vi "TestAddConpane.vi"() -> ()   [LabVIEW 2015]
uses:
  <vilib>/Utility/miscctls.llb/LVPositionTypeDef.ctl
panel:
  in  "E F":dbl
  in  "E":dbl
  in  "D":dbl
  in  "C":dbl
  in  "B":dbl
  in  "A":dbl
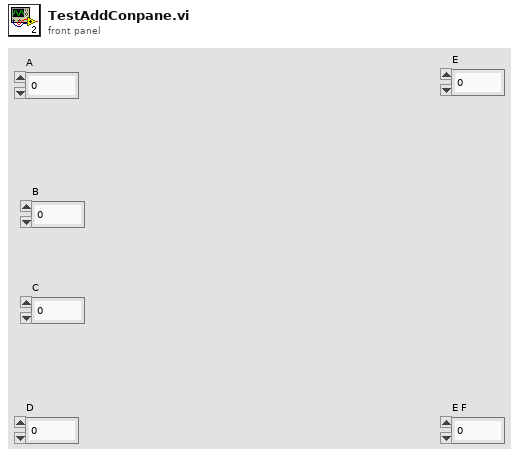
[diagram p1: front panel]
types:
  T1 = cluster{"Left":i32, "Right":i32, "Up":i32, "Down":i32}
  T2 = typedef "LVPositionTypeDef.ctl" = cluster{"Left":i32, "Top":i32}
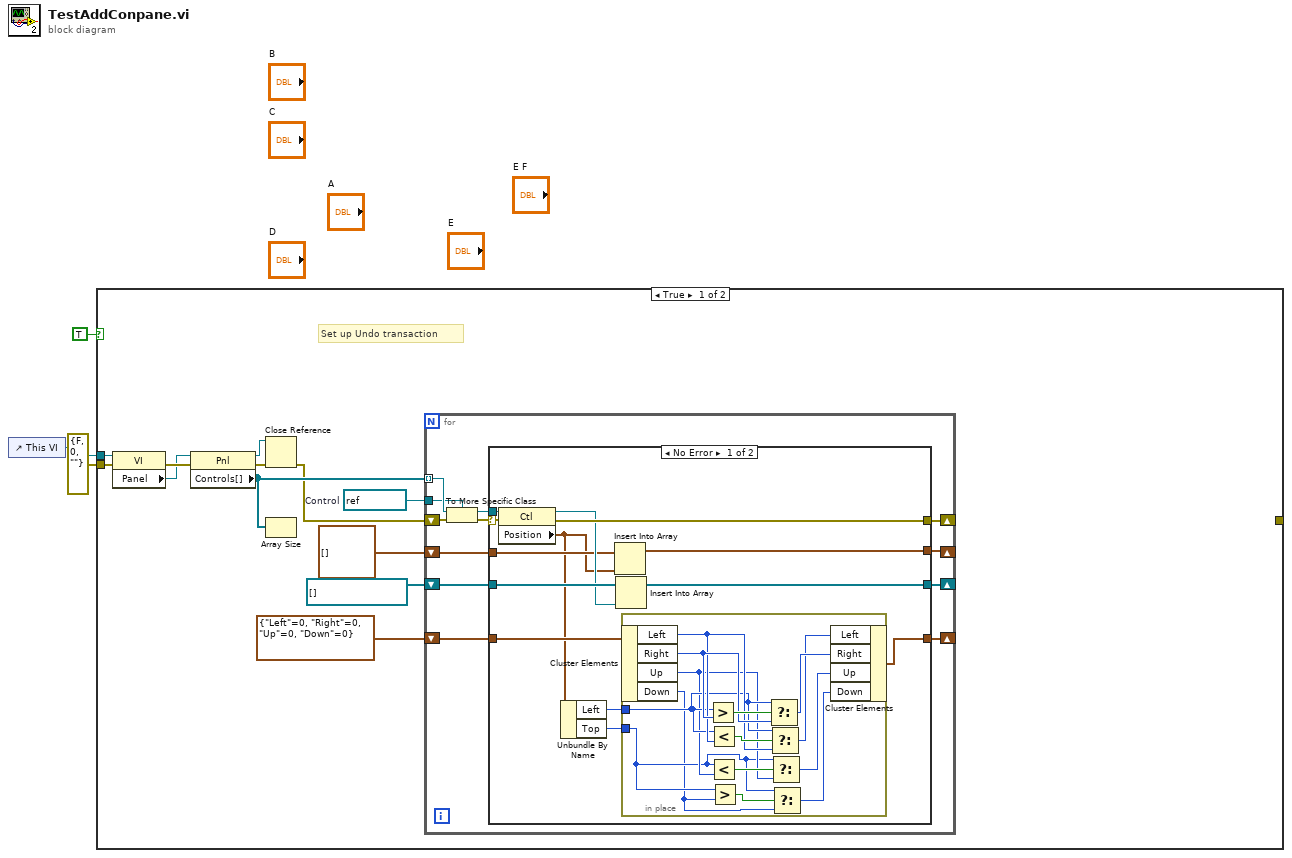
[diagram p0: block diagram]
diagram:
  n1 = control-ref of="This VI"() -> (w3:refnum<vi>)
  n2 = case shown="True" TRUE {
    tunnel: errorcluster {"status"=FALSE, "code"=0, "source"=""} ("error out") -> [w15 w59]
    tunnel: w3 -> [w14 _]
    tunnel: [_ w59] -> _
    frame True {
      w8 = refnum<vi> refnum  # Control
      # "Set up Undo transaction"
      n3 = property class="VI"(reference=w14, error in=w15) -> (error out=w13:errorcluster, "Panel"=w12:refnum<vi>)  [unwired: 1 out]
      n4 = property class="Pnl"(reference=w12, error in=w13) -> (reference out=w11:refnum<vi>, error out=w10:errorcluster, "Controls[]"=w9:refnum<vi>[])
      n5 = Close Reference(reference=w11, error in (no error)=w10) -> (error out=w7:errorcluster)
      n6 = Array Size(array=w9) -> ()  [unwired: 1 out]
      n7 = for {
        tunnel: w9 -> [w27] mode=indexing
        tunnel: w8 -> [w26]
        shift-right: [w21] -> _
        shift-left: refnum<vi>[] [] -> [w22]
        shift-right: [w20] -> _
        shift-left: w7 -> [w25]
        shift-right: [w18] -> _
        shift-left: T2[] [] ("Array") -> [w19]
        shift-right: [w16] -> _
        shift-left: T1 {"Left"=0, "Right"=0, "Up"=0, "Down"=0} -> [w17]
        n8 = To More Specific Class(target class=w26, reference=w27, error in=w25) -> (specific class reference=w23:refnum<vi>, error out=w24:errorcluster)
        n9 = case shown="No Error" w24 {
          selector: w24 -> [w40 w57]
          tunnel: w23 -> [w39 _]
          tunnel: [w38 w57] -> w20
          tunnel: w22 -> [w37 w58]
          tunnel: [w35 w58] -> w21
          tunnel: w19 -> [w34 w56]
          tunnel: [w33 w56] -> w18
          tunnel: w17 -> [w32 w55]
          tunnel: [w28 w55] -> w16
          frame No Error {
            n10 = property class="Ctl"(reference=w39, error in=w40) -> (reference out=w36:refnum<vi>, error out=w38:errorcluster, "Position"=w31:T2)
            n11 = Unbundle By Name(w31) -> ("Left"=w29:i32, "Top"=w30:i32)
            n12 = Insert Into Array(array=w34, new element=w31) -> (w33:T2[])  [unwired: 1 in]
            n13 = Insert Into Array(array=w37, new element=w36) -> (w35:refnum<vi>[])  [unwired: 1 in]
            n14 = in-place {
              in-place-border: w29 -> [w49]
              in-place-border: w30 -> [w43]
              n15 = in-place-cluster #1(w32) -> ("Left"=w50:i32, "Right"=w53:i32, "Up"=w46:i32, "Down"=w42:i32)
              n16 = Greater?(x=w49, y=w53) -> (0:w54:bool)
              n17 = Less?(x=w49, y=w50) -> (x < y?=w51:bool)
              n18 = Less?(x=w43, y=w46) -> (x < y?=w47:bool)
              n19 = Greater?(x=w43, y=w42) -> (0:w44:bool)
              n20 = Select(t=w49, s=w54, f=w53) -> (s? t:f=w52:i32)
              n21 = Select(t=w49, s=w51, f=w50) -> (s? t:f=w48:i32)
              n22 = Select(t=w43, s=w47, f=w46) -> (s? t:f=w45:i32)
              n23 = Select(t=w43, s=w44, f=w42) -> (s? t:f=w41:i32)
              n24 = in-place-cluster #1("Left"=w48, "Right"=w52, "Up"=w45, "Down"=w41) -> (w28:T1)
            }
          }
          frame Error {
          }
        }
      }
    }
    frame False {
      # "Block Diagram"
    }
  }
